vi "FillFGVHDTtransfer.vi"(9 "hdt.int.s.transferSource":u8, 10 "Used":bool, 11 "VI in":refnum<vi>) -> ()   [LabVIEW 2016]
uses:
  controls/Enum.ctl
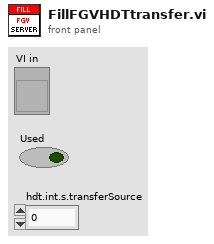
[diagram p1: front panel]
types:
  T1 = typedef "Enum.ctl" = enum16{"Init", "Read", "Write"}
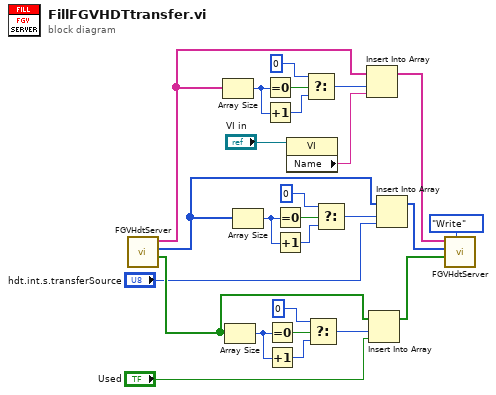
[diagram p0: block diagram]
diagram:
  n1 = call "FGVHdtServer.vi"() -> ("UsedOut"=w24:bool[], "HdtTransferSourceOut"=w3:u8[], "OwnerViOut"=w16:string[])  [unwired: 8 in, 1 out]
  n2 = Array Size(array=w16) -> (size(s)=w15:i32)
  n3 = Array Size(array=w24) -> (size(s)=w19:i32)
  n4 = Array Size(array=w3) -> (size(s)=w5:i32)
  n5 = Equal To 0?(x=w15) -> (x = 0?=w11:bool)
  n6 = Increment(x=w15) -> (x+1=w14:i32)
  n7 = Equal To 0?(x=w19) -> (x = 0?=w23:bool)
  n8 = Increment(x=w19) -> (x+1=w20:i32)
  n9 = Equal To 0?(x=w5) -> (x = 0?=w8:bool)
  n10 = Increment(x=w5) -> (x+1=w6:i32)
  n11 = property class="VI"(reference="VI in") -> ("Name"=w17:string)  [unwired: 1 in, 2 out]
  n12 = Select(t=0, s=w11, f=w14) -> (s? t:f=w13:i32)
  n13 = Select(t=0, s=w23, f=w20) -> (s? t:f=w21:i32)
  n14 = Select(t=0, s=w8, f=w6) -> (s? t:f=w4:i32)
  n15 = Insert Into Array(array=w16, index=w13, new element=w17) -> (w18:string[])
  n16 = Insert Into Array(array=w24, index=w21, new element="Used") -> (w26:bool[])
  n17 = Insert Into Array(array=w3, index=w4, new element="hdt.int.s.transferSource") -> (w1:u8[])
  n18 = call "FGVHdtServer.vi"("Enum"=Enum."Write", "UsedIn"=w26, "HDTTransferSourceIn"=w1, "OwnerViIn"=w18) -> ()  [unwired: 4 in, 4 out]
